vi "PH_AWG-510.Evt Call Set Trigger Settings.vi"(0 "i ref in":refnum<vi>, 1 "Instance":string, 2 "Wanted Trigger Settings":T1, 5 "error in":errorcluster) -> (14 "i ref out":refnum<vi>, 19 "error out":errorcluster)   [LabVIEW 2014, in "PH_AWG-510.lvlib"]
doc: "This VI calls a method by a simple call."
uses:
  PH_AWG-510.lvlib
  PH_AWG-510.Trigger Settings.ctl
  CS_Core/CSSystem/CoreLib/CoreLib.short 2 byte array.vi
  CS_Core/CSSystem/CoreLib/CoreLib.double 2 byte array.vi
  CS_Core/CSSystem/CoreLib/CoreLib.lvlib
  CS_Core/BaseProcess/BaseProcess.lvlib
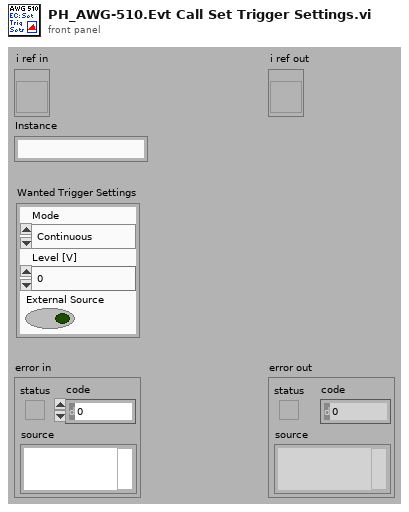
[diagram p1: front panel]
types:
  T1 = typedef "PH_AWG-510.lvlib/PH_AWG-510.Trigger Settings.ctl" = cluster{"Mode":enum16{"Continuous", "Triggered", "Gated", "Enhanced"}, "Level (V)":dbl, "External Source":bool}
  T2 = enum16{"Continuous", "Triggered", "Gated", "Enhanced"}
  T3 = typedef "CoreDefs.rawDataType.ctl" = i8[]
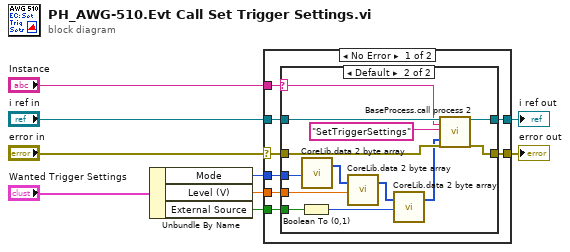
[diagram p0: block diagram]
diagram:
  n1 = Unbundle By Name("Wanted Trigger Settings") -> ("Mode"=w3:T2, "Level (V)"=w2:dbl, "External Source"=w1:bool)
  n2 = case shown="No Error" "error in" {
    selector: "error in" -> [w13 w33]
    tunnel: [w17 w33] -> w6
    tunnel: "Instance" -> [w12 _]
    tunnel: "i ref in" -> [w16 w34]
    tunnel: [w15 w34] -> w8
    tunnel: w3 -> [w14 _]
    tunnel: w1 -> [w11 _]
    tunnel: w2 -> [w10 _]
    frame No Error {
      n3 = case shown="Default" w12 {
        selector: w12 -> [_ w22]
        tunnel: [w19 w32] -> w17
        tunnel: w13 -> [w19 w30]
        tunnel: w16 -> [w18 w29]
        tunnel: [w18 w28] -> w15
        tunnel: w14 -> [_ w27]
        tunnel: w11 -> [_ w21]
        tunnel: w10 -> [_ w24]
        frame "", "N/A" {
        }
        frame Default {
          n4 = Boolean To (0,1)(Boolean=w21) -> (0, 1=w20:i16)
          n5 = call-poly "CoreLib.data 2 byte array.vi"("i16"=w27) -> ("byteArray out"=w26:T3)  [unwired: 18 in]
          n6 = call-poly "CoreLib.data 2 byte array.vi"("byteArray"=w26, "f64"=w24) -> ("byteArray out"=w25:T3)  [unwired: 17 in]
          n7 = call-poly "CoreLib.data 2 byte array.vi"("byteArray"=w25, "i16"=w20) -> ("byteArray out"=w23:T3)  [unwired: 17 in]
          n8 = call "BaseProcess.call process 2.vi"("i ref in"=w29, "Object"=w22, "Selector"="SetTriggerSettings", "Data"=w23, "error in (no error)"=w30) -> ("i ref out"=w28:refnum<vi>, "error out"=w32:errorcluster)  [unwired: 13 in]
        }
      }
    }
    frame Error {
    }
  }
  "i ref out" <- w8
  "error out" <- w6
